vi "Topo & GridSpectr_DriftCorrection_v12.vi"(6 "Internal use":string, 7 "Grid param":T1 {"height (m)" format="%#_6p"; "width (m)" format="%#_6p"; "center Y (m)" format="%#_6p"; "center X (m)" format="%#_6p"}, 8 "Error in (no error)":errorcluster, 9 "Points Y/Index Y":i32, 10 "Points X/Index X":i32, 11 "Method":enum16{"init", "run", "end"}(ring)=enum."end") -> (0 "Error out":errorcluster)   [LabVIEW 2014]
doc: "Example of a measurement VI to be used in the \"Experiments on a Grid\" tool as external VI.\n\nThis example measure the topography and spectroscopy data. The spectroscopy measurements are taken on a subgrid. The data are saved to a sxm and a binary file.\n\n- Nanonis Programming Interface -"
uses:
  <userlib>/Nanonis Prog Interface V5/Scan/Grid/LinePatternGet.vi
  <userlib>/Nanonis Prog Interface V5/Scan/Grid/GridPatternGet.vi
  <userlib>/Nanonis Prog Interface V5/Scan/Grid/CloudPatternGet.vi
  <userlib>/Nanonis Prog Interface V5/Nanonis Prog Interface.lvlib
panel:
  in  "type":u16(ring)=1 items=["Line", "Grid", "Cloud"]
  in  "Lockin ON/OFF":bool
  in  "Correct Drift":bool=TRUE
  in  "Email when finished":string="cornelius.krull@monash.edu, dhaneesh.gopalakrishnan@monash.edu"
  in  "STS z offset":dbl format="%#_6p"
  out "ETA":timestamp=timestamp(3582621546.85837 s since 1904-01-01)
  out "remaining":dbl=19834.093046092985 format="%<%H:%M:%S>t"
  out "Progress":u8(slide)=5 scale=0.0..100.0 scale format="%#.1g"
  out "total Points":i32=576
  in  "preSTS delay [ms]":u32=3
  in  "STS Bias":dbl=-3.4 format="%#_6p"
  in  "Move Bias":dbl=-3.4 format="%#_6p"
  in  "Move Current":dbl=5e-11 format="%#_6p"
  in  "Imaging Bias":dbl=-3.4 format="%#_6p"
  in  "max applied Drift Correction":i32=20 min=1 max=100 step=1 format="%.0p"
  in  "Correlate":u16(ring) items=["first Frame", "successive Frames"]
  out "Topo Images taken":i32
  in  "Increment":i32=40
  in  "Threshold":i32=2 min=1 step=1
  in  "tip Speed (m/s)":sgl=1e-08 format="%.2p"
  out "X drift":i32
  out "Y drift":i32
  out "Last Drift detected":i32
  in  "MaxImagesBack":i32=2
  in  "Channel index (0-23)":u8(ring) items=["Current"=0, "Z (m)"=14]
  in  "File name":string="DCA_cluster_STS_Grid"
  in  "STS Current":dbl=5e-11 format="%#_6p"
  in  "Imaging Current":dbl=5e-11 format="%#_6p"
  in  "zdrift \nDuration (s)":dbl
  in  "Correct z drift":bool
  out "Status":string="finishing"
  in  "Drift correction Pixels":i32=256 caption="Topo Pixels"
  out "Y Offset":dbl format="%#_6p"
  out "X Offset":dbl format="%#_6p"
  out "Points taken":dbl=30.0
  in  "Drift Correction every":i32=40
  in  "Y subgrid spacing":u16=1
  in  "X subgrid spacing":u16=1
  # "GRID points"
  # "Increase this if no Drift was detected for \na certain number of images"
  # "%"
  # "time (HH:MM:SS)"
  # "images back"
  # "% of image size"
  # "RUN smart tilt before starting the GRID | Img Angle = 0"
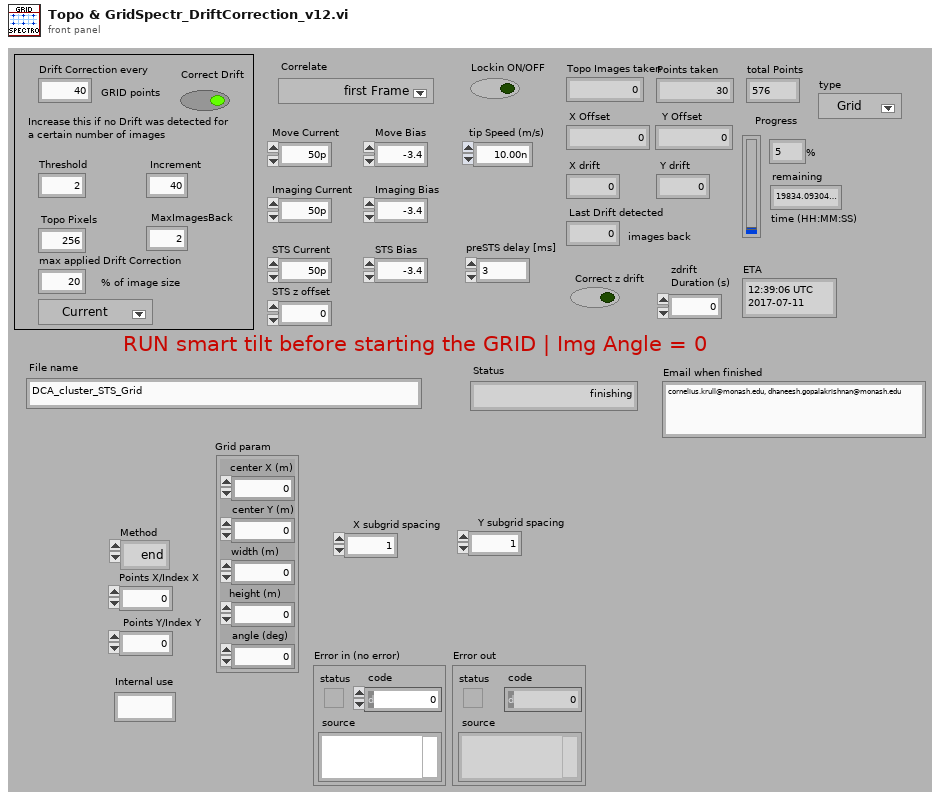
[diagram p1: front panel]
types:
  T1 = cluster{"center X (m)":sgl, "center Y (m)":sgl, "width (m)":sgl, "height (m)":sgl, "angle (deg)":sgl}
  T2 = cluster{"Drift correction Pixels":i32, "Imaging Current":dbl, "STS Current":dbl, "MaxImagesBack":i32, "tip Speed (m/s)":sgl, "Threshold":i32, "Increment":i32, "Correlate":u16, "max applied Drift Correction":i32, "Imaging Bias":dbl, "Move Current":dbl, "Move Bias":dbl, "STS Bias":dbl, "preSTS delay [ms]":u32, "STS z offset":dbl, "Correct Drift":bool, "Lockin ON/OFF":bool}
  T3 = cluster{"center X":sgl, "center Y":sgl, "angle":sgl, "width":sgl, "height":sgl, "# pixels":i32, "# lines":i32}
  T4 = cluster{"Name":string, "Calibration":sgl, "Offset":sgl, "Channel index":i32}[]
  T5 = cluster{"up/down":bool, "time/line":sgl, "start time":timestamp, "end time":timestamp}
  T6 = cluster{"Z averaging time (s)":sgl, "Z offset (m)":sgl, "Initial settling time (s)":sgl}
  T7 = cluster{"Max. slew rate (V/s)":sgl, "Settling time (s)":sgl, "Integration time (s)":sgl}
  T8 = cluster{"End settling time (s)":sgl, "Z control time (s)":sgl}
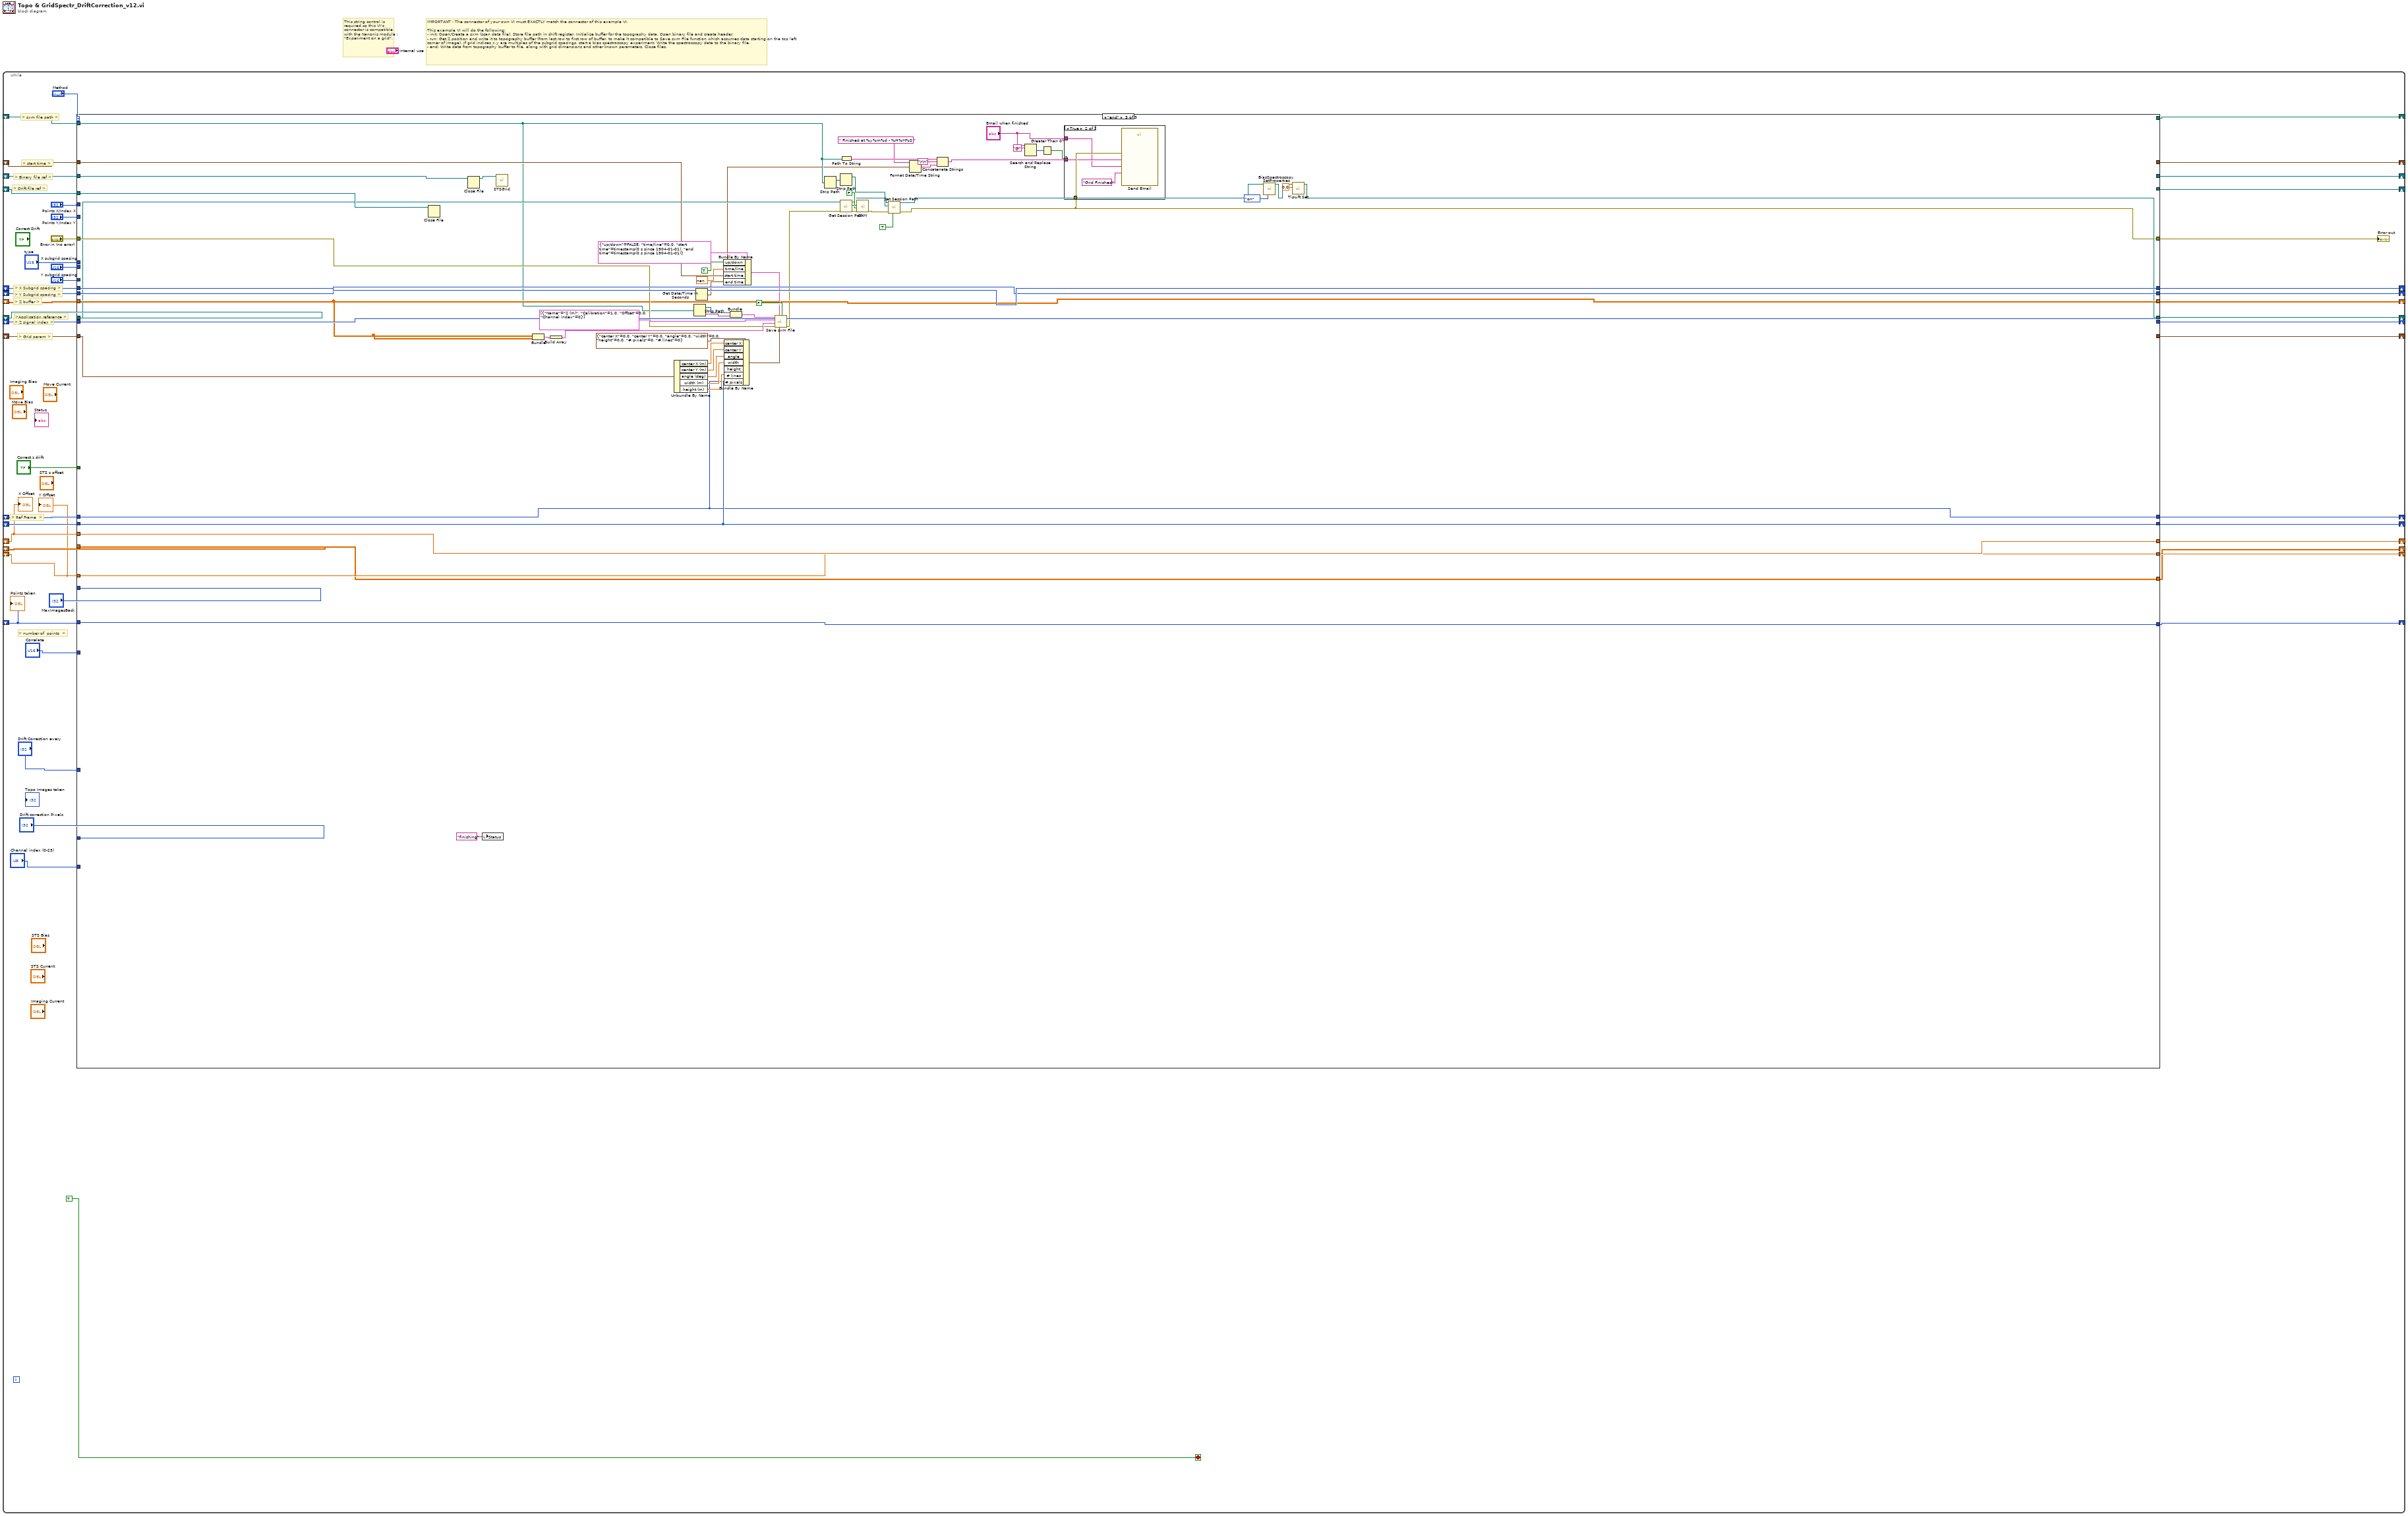
[diagram p0: block diagram]
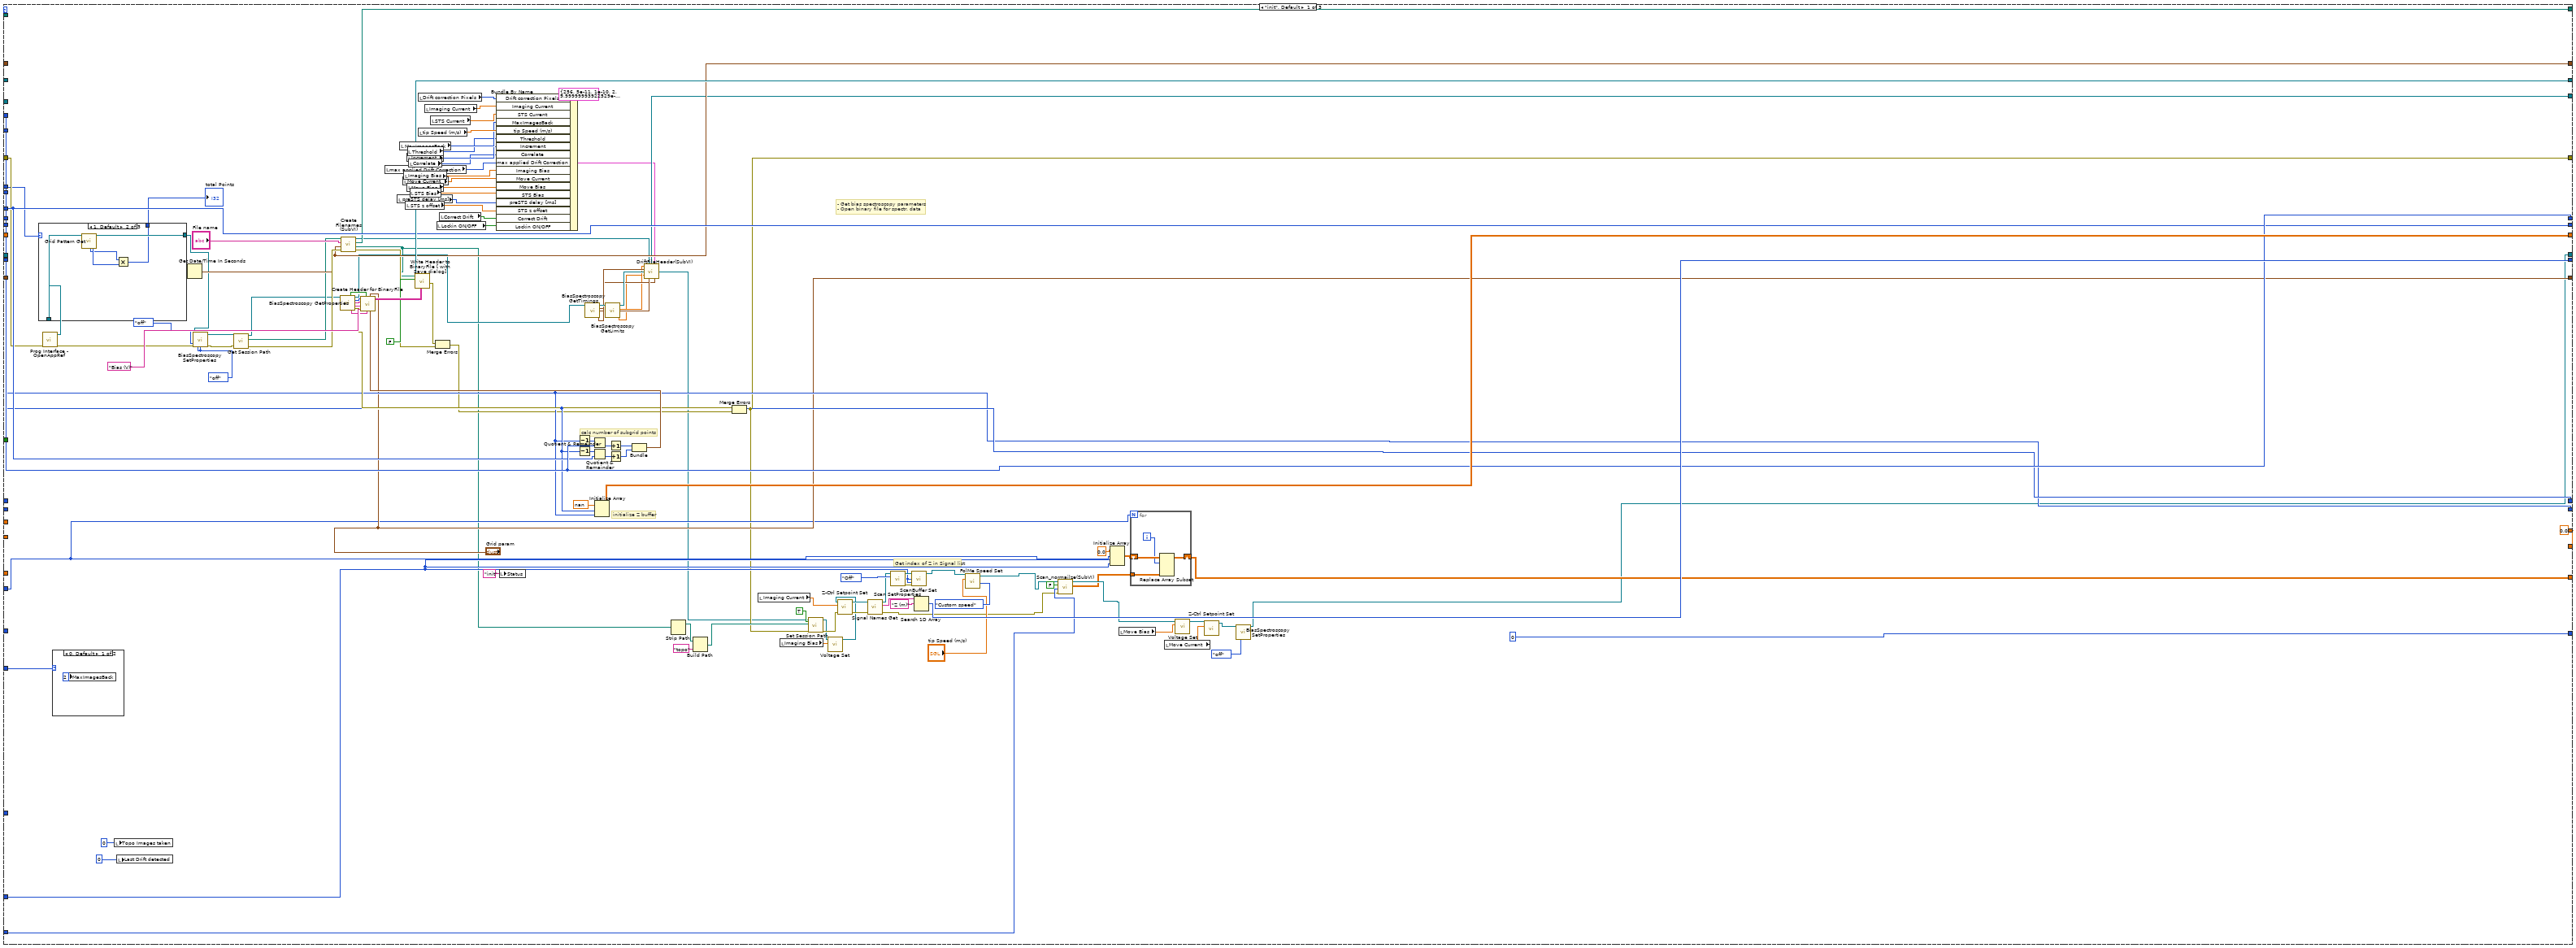
[diagram p2: hidden frame]
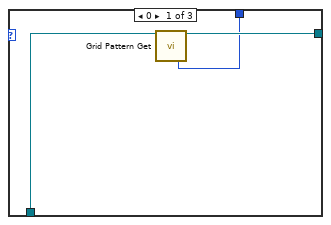
[diagram p3: hidden frame]
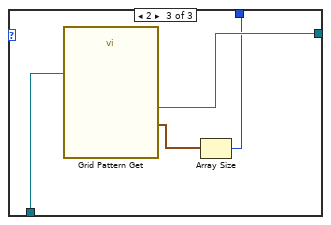
[diagram p4: hidden frame]
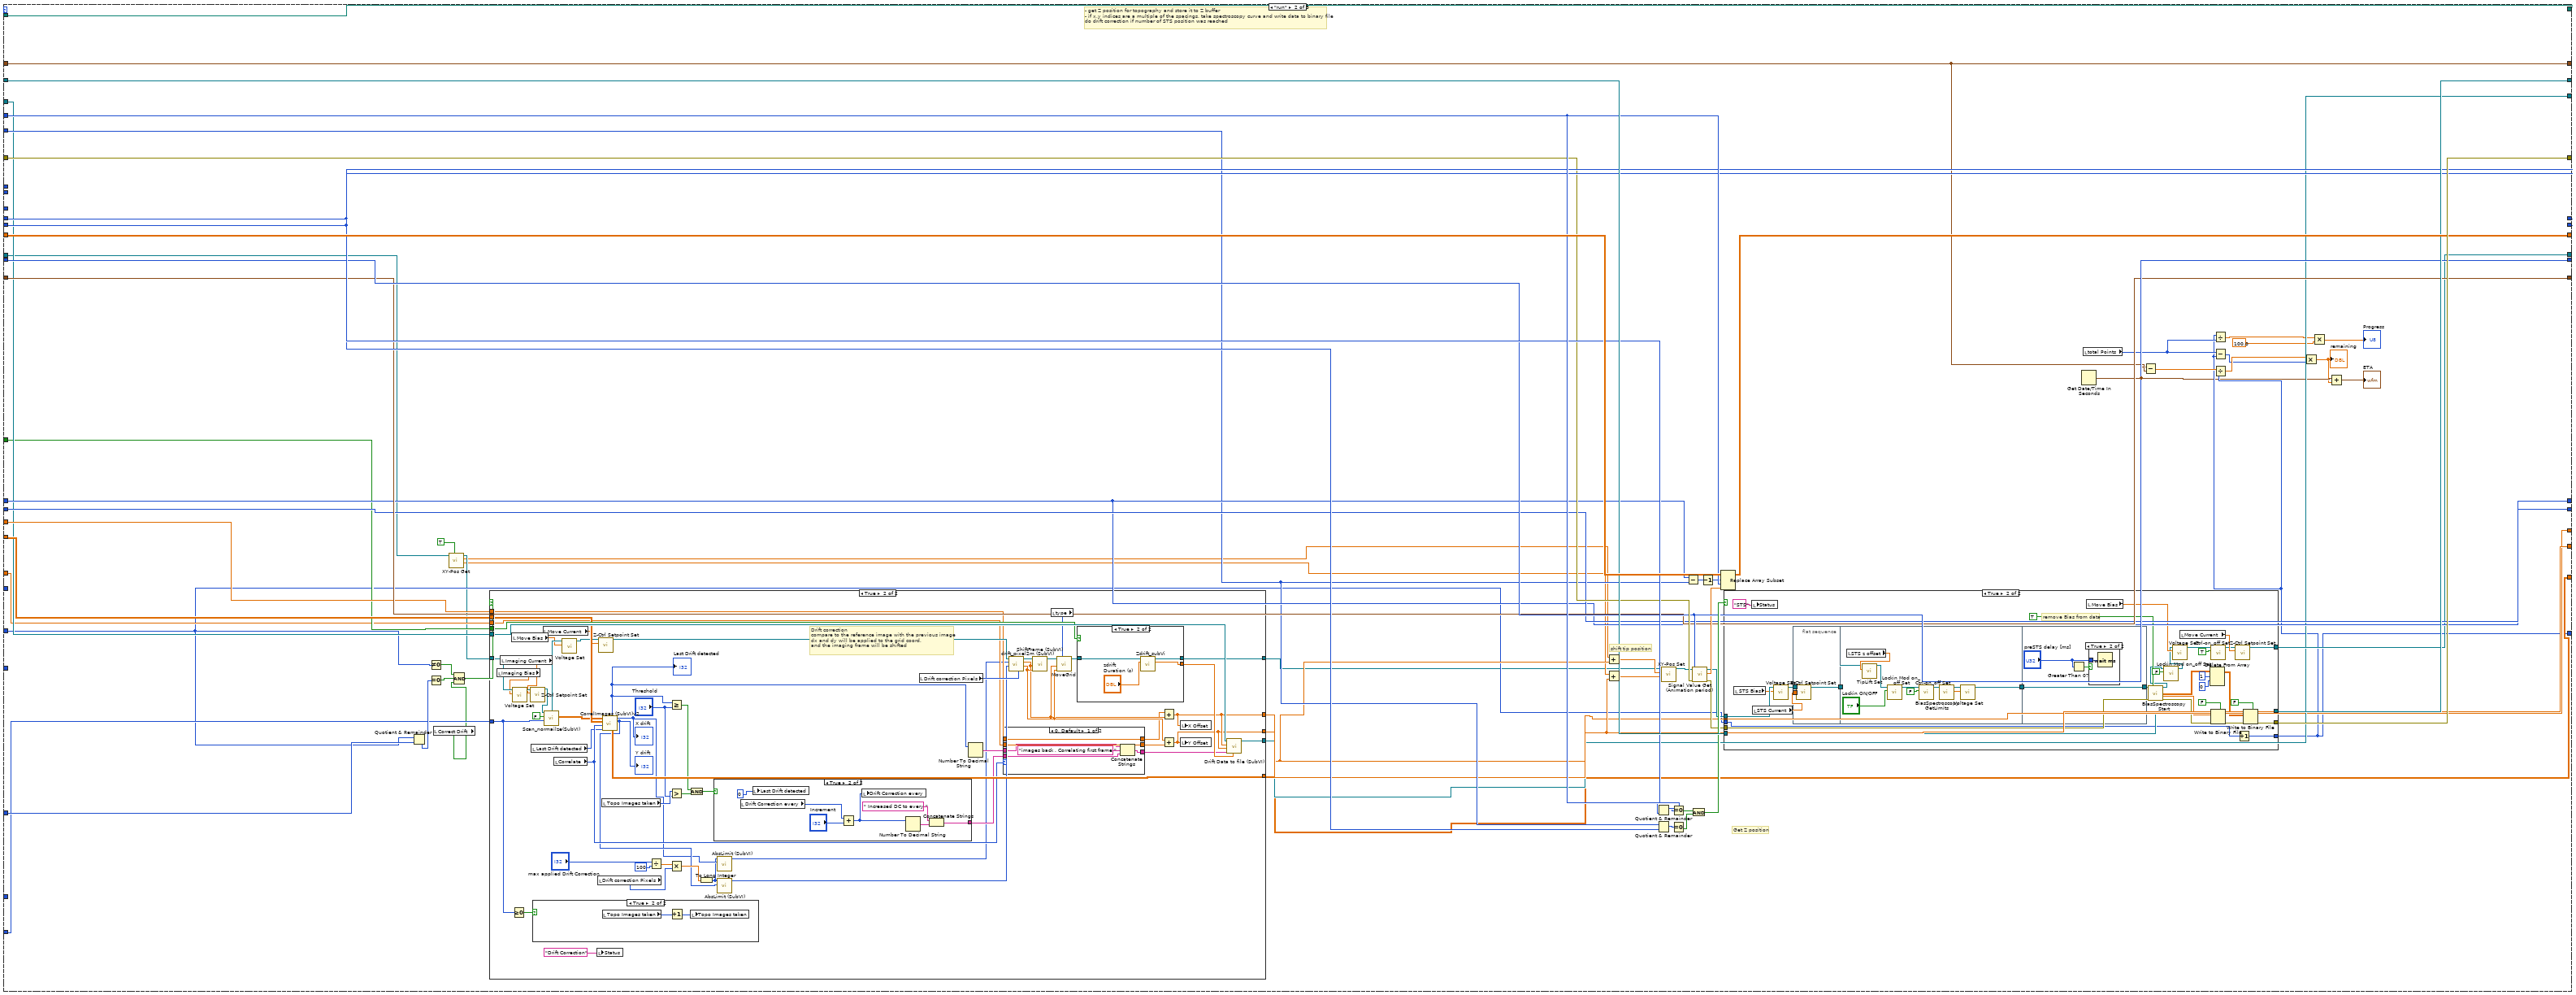
[diagram p6: hidden frame]
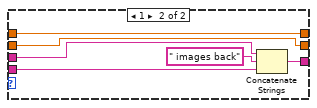
[diagram p8: hidden frame]
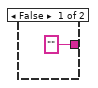
[diagram p10: hidden frame]
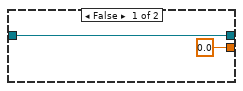
[diagram p11: hidden frame]
diagram:
  # "This string control is required so this VI's connector is compatible with the Nanonis module : \"Experiment on a grid\"."
  # "IMPORTANT : The connector of your own VI must EXACTLY match the connector of this example VI.\n\nThis example VI will do the following:\n- init: Open/Create a sxm (scan data file). Store file path in shift register. Initialize buffer for the topography data. Open binary file and create header.\n- run: Get Z position and write it to topography buffer (from last row to first row of buffer, to make it compatible to Save sxm File function which assumes data starting on the top left corner of image). If grid indices x,y are multiples of the subgrid spacings, start a bias spectroscopy experiment. Write the spectroscopy data to the binary file.\n- end: Write data from topography buffer to file, along with grid dimensions and other known parameters. Close files."
  n1 = while {
    shift-right: [w22] -> _
    shift-left: _ -> [w45]
    shift-right: [w40] -> _
    shift-left: _ -> [w39]
    shift-right: [w37] -> _
    shift-left: _ -> [w38]
    shift-right: [w36] -> _
    shift-left: _ -> [w35]
    shift-right: [w29] -> _
    shift-left: _ -> [w31]
    shift-right: [w30] -> _
    shift-left: _ -> [w32]
    shift-right: [w28] -> _
    shift-left: _ -> [w27]
    shift-right: [w26] -> _
    shift-left: _ -> [w25]
    shift-right: [w24] -> _
    shift-left: _ -> [w23]
    shift-right: [w21] -> _
    shift-left: _ -> [w20]
    shift-right: [w19] -> _
    shift-left: _ -> [w18]
    shift-right: [w17] -> _
    shift-left: _ -> [w10]
    shift-right: [w16] -> _
    shift-left: _ -> [w9]
    shift-right: [w15] -> _
    shift-left: _ -> [w12]
    shift-right: [w14] -> _
    shift-left: _ -> [w11]
    shift-right: [w7] -> _
    shift-left: _ -> [w6]
    stop <- TRUE stop-if-true
    # "> Drift file ref >"
    # "> number of  points  >"
    # "> Ref Frame  >"
    # "> Grid param >"
    # "> start time >"
    # ">Application reference >"
    # "> Y Subgrid spacing >"
    # "> X Subgrid spacing >"
    # "> Z signal index >"
    # "> Binary file ref >"
    # "> Z buffer >"
    # "> sxm file path >"
    n2 = case shown="\"end\"" "Method" {
      tunnel: [w128 w247 _] -> w22
      tunnel: w45 -> [_ w247 w412]
      tunnel: "Error in (no error)" -> [w130 w233 w439]
      tunnel: [w52 w246 w394] -> w43
      tunnel: "Points X/Index X" -> [w142 w241 _]
      tunnel: "Points Y/Index Y" -> [w143 w226 _]
      tunnel: [w166 w244 w428] -> w40
      tunnel: w39 -> [_ w245 w428]
      tunnel: w38 -> [_ w243 w421]
      tunnel: [w158 w242 _] -> w37
      tunnel: [w156 w231 w453] -> w36
      tunnel: w35 -> [_ w231 w453]
      tunnel: "X subgrid spacing" -> [w155 _ _]
      tunnel: "Y subgrid spacing" -> [w154 _ _]
      tunnel: w32 -> [_ w235 w452]
      tunnel: w31 -> [_ w234 w451]
      tunnel: [w155 w235 w452] -> w30
      tunnel: [w154 w234 w451] -> w29
      tunnel: [w92 w219 w399] -> w28
      tunnel: w27 -> [_ w202 w416]
      tunnel: ["Grid param" w229 _] -> w26
      tunnel: w25 -> [_ w229 w438]
      tunnel: [w127 w192 _] -> w24
      tunnel: w23 -> [_ w192 w446]
      tunnel: [w143 w227 w429] -> w21
      tunnel: w20 -> [_ w227 w429]
      tunnel: [w142 w228 w430] -> w19
      tunnel: w18 -> [_ w228 w430]
      tunnel: [w139 w209 w427] -> w17
      tunnel: [w139 w214 w425] -> w16
      tunnel: [w123 w208 w422] -> w15
      tunnel: [0 w190 w426] -> w14
      tunnel: w11 -> [_ w205 w426]
      tunnel: "Drift Correction every" -> [_ w222 _]
      tunnel: w12 -> [_ w213 w422]
      tunnel: w10 -> [_ w220 w427]
      tunnel: w9 -> [_ w206 w425]
      tunnel: "Drift correction Pixels" -> [w122 _ _]
      tunnel: [w87 w211 _] -> w7
      tunnel: w6 -> [_ w212 w423]
      tunnel: "Correct z drift" -> [_ w210 _]
      tunnel: "Channel index (0-23)" -> [w61 w207 _]
      tunnel: "MaxImagesBack" -> [w121 _ _]
      tunnel: "Correlate" -> [w103 _ _]
      tunnel: "type" -> [w55 _ _]
      frame "init", Default {
        w89 = enum16{"no change", "on", "off"}."off" ("Save dialog")
        w139 = 0.0
        # "- Get bias spectroscopy parameters\n- Open binary file for spectr. data"
        # "initialize Z buffer"
        # "calc number of subgrid points"
        # "Get index of Z in Signal list"
        n3 = call <userlib>:"Prog Interface - OpenAppRef.vi"("Error in (no error)"=w130) -> ("Error out"=w109:errorcluster, "Application reference"=w94:refnum<vi>)  [unwired: 5 in]
        n4 = case shown="1, Default" w55 {
          tunnel: w94 -> [w169 w174 w178]
          tunnel: [w168 w173 w177] -> w93
          tunnel: [w167 w170 w175] -> w54
          frame 0 {
            n5 = call-poly <userlib>:"Grid Pattern Get.vi"("Application ref in"=w169) -> ("Points"=w167:i32, "Application ref out"=w168:refnum<vi>)  [unwired: 12 in, 5 out]
          }
          frame 1, Default {
            n6 = call-poly <userlib>:"Grid Pattern Get.vi"("Application ref in"=w174) -> ("Points Y"=w171:i32, "Points X"=w172:i32, "Application ref out"=w173:refnum<vi>)  [unwired: 10 in, 6 out]
            n7 = Multiply(x=w171, y=w172) -> (x*y=w170:i32)
          }
          frame 2 {
            n8 = call-poly <userlib>:"Grid Pattern Get.vi"("Application ref in"=w178) -> ("Application ref out"=w177:refnum<vi>, "Cloud data"=w176:cluster{"X":sgl, "Y":sgl}[])  [unwired: 16 in, 1 out]
            n9 = Array Size(array=w176) -> (size(s)=w175:i32)
          }
        }
        "total Points" <- w54
        n10 = case shown="0, Default" w103 {
          frame 0, Default {
            n11 = local write "MaxImagesBack"(2 ("StepsBack")) -> ()
          }
          frame 1 {
          }
        }
        n12 = local write "Topo Images taken"(0 ("Images taken")) -> ()
        n13 = local write "Last Drift detected"(0 ("Last Drift detected")) -> ()
        n14 = Get Date/Time In Seconds() -> (seconds since 1Jan1904=w127:timestamp)
        n15 = call <userlib>:"BiasSpectroscopy SetProperties.vi"("Application ref in"=w93, "Autosave (no change)"=enum16{"no change", "on", "off"}."off", "Error in (no error)"=w109, "Z-Controller hold (no change)"=w89, "Save dialog"=w89) -> ("Application ref out"=w106:refnum<vi>, "Error out"=w105:errorcluster)  [unwired: 9 in]
        n16 = call <userlib>:"Get Session Path.vi"("error in (no error)"=w105, "Application ref in"=w106) -> ("error out"=w129:errorcluster, "Session path"=w113:path, "Application ref out"=w107:refnum<vi>)  [unwired: 7 in]
        n17 = call <userlib>:"BiasSpectroscopy GetProperties.vi"("Application ref in"=w107) -> ("Backward sweep"=w162:bool, "Application ref out"=w116:refnum<vi>, "Number of points"=w145:i32, "Channels"=w144:string[], "Parameters"=w160:string[], "Fixed parameters"=w147:string[], "Error out"=w159:errorcluster)  [unwired: 6 in, 2 out]
        n18 = call "Create Filenames (SubVI).vi"("error in (no error)"=w129, "seconds since 1Jan1904"=w127, "File name"="File name", "Session path"=w113) -> ("error out"=w117:errorcluster, "binFilePath"=w110:path, "topoFilePath"=w128:path, "Drift File out"=w88:refnum<file>)  [unwired: 4 in]
        n19 = local read "max applied Drift Correction"() -> (w69:i32)
        n20 = local read "preSTS delay [ms]"() -> (w64:u32)
        n21 = local read "MaxImagesBack"() -> (w73:i32)
        n22 = local read "Move Current"() -> (w67:dbl)
        n23 = local read "Imaging Bias"() -> (w68:dbl)
        n24 = local read "STS z offset"() -> (w63:dbl)
        n25 = local read "Increment"() -> (w71:i32)
        n26 = local read "Move Bias"() -> (w66:dbl)
        n27 = local read "Threshold"() -> (w72:i32)
        n28 = local read "Correlate"() -> (w70:u16)
        n29 = local read "STS Bias"() -> (w65:dbl)
        n30 = local read "Drift correction Pixels"() -> (w78:i32)
        n31 = local read "tip Speed (m/s)"() -> (w75:sgl)
        n32 = local read "Imaging Current"() -> (w77:dbl)
        n33 = local read "STS Current"() -> (w76:dbl)
        n34 = local read "Lockin ON/OFF"() -> (w74:bool)
        n35 = local read "Correct Drift"() -> (w62:bool)
        n36 = Bundle By Name(cluster=T2 {"Drift correction Pixels"=256, "Imaging Current"=5e-11, "STS Current"=1e-10, "MaxImagesBack"=2, "tip Speed (m/s)"=1e-08, "Threshold"=2, "Increment"=64, "Correlate"=0, "max applied Drift Correction"=20, "Imaging Bias"=-0.02, "Move Current"=1.5e-11, "Move Bias"=-0.02, "STS Bias"=0.1, "preSTS delay [ms]"=1000, "STS z offset"=-1.7e-10, "Correct Drift"=TRUE, "Lockin ON/OFF"=TRUE} ("Drift Correction"), "Drift correction Pixels"=w78, "Imaging Current"=w77, "STS Current"=w76, "MaxImagesBack"=w73, "tip Speed (m/s)"=w75, "Threshold"=w72, "Increment"=w71, "Correlate"=w70, "max applied Drift Correction"=w69, "Imaging Bias"=w68, "Move Current"=w67, "Move Bias"=w66, "STS Bias"=w65, "preSTS delay [ms]"=w64, "STS z offset"=w63, "Correct Drift"=w62, "Lockin ON/OFF"=w74) -> (w80:T2)
        n37 = local write "Status"("init" ("Status")) -> ()
        n38 = Decrement(x=w142) -> (x-1=w153:i32)
        n39 = Decrement(x=w143) -> (x-1=w152:i32)
        n40 = call <userlib>:"BiasSpectroscopy GetTimings.vi"("Application ref in"=w116) -> ("Application ref out"=w120:refnum<vi>, "Initialization"=w83:T6, "Sweep Timing"=w84:T7, "End of Sweep"=w85:T8)  [unwired: 10 in, 1 out]
        n41 = Quotient & Remainder(x=w153, y=w155) -> (floor(x/y)=w151:i32)  [unwired: 1 out]
        n42 = Quotient & Remainder(x=w152, y=w154) -> (floor(x/y)=w150:i32)  [unwired: 1 out]
        n43 = Initialize Array(sgl nan ("element"), w143, w142) -> (w166:sgl[][])
        n44 = call <userlib>:"BiasSpectroscopy GetLimits.vi"("Application ref in"=w120) -> ("End value (V)"=w81:sgl, "Start value (V)"=w82:sgl, "Application ref out"=w86:refnum<vi>)  [unwired: 5 in, 1 out]
        n45 = Increment(x=w151) -> (x+1=w149:i32)
        n46 = Increment(x=w150) -> (x+1=w148:i32)
        n47 = Bundle(w149, w148) -> (w161:cluster{i32, i32})  [unwired: 1 in]
        n48 = call <userlib>:"Create Header for BinaryFile.vi"("Grid points"=w161, "Grid param"="Grid param", "Fixed parameters"=w147, "Backward sweep"=w162, "Sweep signal"="Bias (V)" ("Sweep Signal"), "Parameters"=w160, "Channels"=w144, "Points per sweep"=w145) -> ("Header (fixed attributes)"=w164:string[][])  [unwired: 3 in]
        n49 = call <userlib>:"Write Header to BinaryFile [ with Save dialog].vi"("Fixed Attributes"=w164, "Show Dialog? (T)"=FALSE, "Filename"=w110) -> ("Error out"=w118:errorcluster, "File ref"=w158:refnum<file>)  [unwired: 5 in, 2 out]
        n50 = Merge Errors(w118, w117) -> (w119:errorcluster)
        n51 = call "DriftFileHeader(SubVI).vi"("Start value (V)"=w82, "Byte Stream File in"=w88, "Drift Correction"=w80, "End of Sweep"=w85, "Application ref in"=w86, "End value (V)"=w81, "Sweep Timing"=w84, "Initialization"=w83) -> ("Byte Stream File out"=w87:refnum<file>, "Application ref out"=w49:refnum<vi>)  [unwired: 6 in]
        n52 = Strip Path(path=w110) -> (stripped path=w112:path)  [unwired: 1 out]
        n53 = Build Path(base path=w112, name or relative path="topo") -> (appended path=w53:path)
        n54 = Merge Errors(w159, w119) -> (w52:errorcluster)
        n55 = local read "Imaging Current"() -> (w95:dbl)
        n56 = local read "Imaging Bias"() -> (w96:dbl)
        n57 = call <userlib>:"Set Session Path.vi"("Save settings to previous? (False)"=TRUE, "error in (no error)"=w52, "Session Folder"=w53, "Application ref in"=w49) -> ("error out"=w51:errorcluster, "Application ref out"=w48:refnum<vi>)  [unwired: 6 in]
        n58 = call <userlib>:"Voltage Set.vi"("Bias (V)"=w96, "Application ref in"=w48) -> ("Application ref out"=w99:refnum<vi>)  [unwired: 8 in, 1 out]
        n59 = call <userlib>:"Z-Ctrl Setpoint Set.vi"("error in (no error)"=w51, "Z Controller setpoint"=w95, "Application ref in"=w99) -> ("error out"=w131:errorcluster, "Application ref out"=w132:refnum<vi>)  [unwired: 7 in]
        n60 = call <userlib>:"Signal Names Get.vi"("error in (no error)"=w131, "Application ref in"=w132) -> ("error out"=w58:errorcluster, "Signals Names"=w146:string[], "Application ref out"=w135:refnum<vi>)  [unwired: 5 in]
        n61 = call <userlib>:"Scan SetProperties.vi"("Application ref in"=w135, "Continuous scan"=enum16{"No change", "On", "Off"}."Off") -> ("Application ref out"=w137:refnum<vi>, "Error out"=w136:errorcluster)  [unwired: 12 in]
        n62 = call <userlib>:"ScanBuffer Set.vi"("Application ref in"=w137, "Pixels"=w122, "Lines"=w122, "error in (no error)"=w136) -> ("Application ref out"=w101:refnum<vi>)  [unwired: 10 in, 1 out]
        n63 = Search 1D Array(1D array=w146, element="Z (m)") -> (index of element=w156:i32)  [unwired: 1 in]
        n64 = call <userlib>:"FolMe Speed Set.vi"("Speed Setting (Custom)"=enum32{"Scan speed", "Custom speed"}."Custom speed", "Speed (m/s)"="tip Speed (m/s)", "Application ref in"=w101) -> ("Application ref out"=w60:refnum<vi>)  [unwired: 5 in, 1 out]
        n65 = call "Scan_normailze(SubVI).vi"("error in (no error)"=w58, "Channel index (0-23)"=w61, "Normalization"=FALSE ("Boolean"), "Application in"=w60) -> ("Array"=w57:dbl[][], "Application out"=w59:refnum<vi>)  [unwired: 5 in, 1 out]
        n66 = Initialize Array(0.0 ("element"), w121, w122, w122) -> (w124:dbl[][][])
        n67 = local read "Move Bias"() -> (w98:dbl)
        n68 = for {
          N: w121 -> [_]
          tunnel: w57 -> [w182]
          shift-right: [w181] -> w123
          shift-left: w124 -> [w183]
          i -> [w180]
          n69 = Replace Array Subset(array=w183, new element=w182, index (dim 0)=w180) -> (w181:dbl[][][])  [unwired: 2 in]
        }
        n70 = local read "Move Current"() -> (w97:dbl)
        n71 = call <userlib>:"Voltage Set.vi"("Bias (V)"=w98, "Application ref in"=w59) -> ("Application ref out"=w100:refnum<vi>)  [unwired: 8 in, 1 out]
        n72 = call <userlib>:"Z-Ctrl Setpoint Set.vi"("Z Controller setpoint"=w97, "Application ref in"=w100) -> ("Application ref out"=w91:refnum<vi>)  [unwired: 8 in, 1 out]
        n73 = call <userlib>:"BiasSpectroscopy SetProperties.vi"("Application ref in"=w91, "Z-Controller hold (no change)"=enum16{"no change", "on", "off"}."off") -> ("Application ref out"=w92:refnum<vi>)  [unwired: 12 in, 1 out]
      }
      frame "run" {
        # "shift tip position"
        # "Get Z position"
        # "- get Z position for topography and store it to Z buffer\n- if x,y indices are a multiple of the spacings, take spectroscopy curve and write data to binary file\ndo drift correction if number of STS position was reached"
        n74 = Quotient & Remainder(x=w205, y=w222) -> (x-y*floor(x/y)=w223:i32)  [unwired: 1 out]
        n75 = Not Equal To 0?(x=w205) -> (x != 0?=w203:bool)
        n76 = Equal To 0?(x=w223) -> (x = 0?=w221:bool)
        n77 = local read "Correct Drift"() -> (w184:bool)
        n78 = call <userlib>:"XY-Pos Get.vi"("Wait for newest data (F=False)"=TRUE, "Application ref in"=w202) -> ("Y (m)"=w198:sgl, "X (m)"=w199:sgl, "Application ref out"=w201:refnum<vi>)  [unwired: 5 in, 1 out]
        n79 = Compound Arithmetic op=AND(w203, w221, w184) -> (w204:bool)
        n80 = case shown="True" w204 {
          tunnel: w201 -> [w252 w262]
          tunnel: [w252 w304] -> w197
          tunnel: w213 -> [w249 w299]
          tunnel: [w251 w302] -> w209
          tunnel: [w250 w301] -> w214
          tunnel: w220 -> [w251 w278]
          tunnel: w206 -> [w250 w276]
          tunnel: [w249 w295] -> w208
          tunnel: w212 -> [w248 w307]
          tunnel: [w248 w306] -> w211
          tunnel: w210 -> [_ w303]
          tunnel: w207 -> [_ w282]
          frame False {
          }
          frame True {
            # "Drift correction \ncompare to the reference image with the previous image \ndx and dy will be applied to the grid coord, \nand the imaging frame will be shifted"
            n81 = local read "Imaging Bias"() -> (w260:dbl)
            n82 = local read "Imaging Current"() -> (w259:dbl)
            n83 = local read "Move Bias"() -> (w256:dbl)
            n84 = Greater Or Equal To 0?(x=w282) -> (x >= 0?=w281:bool)
            n85 = call <userlib>:"Voltage Set.vi"("Bias (V)"=w260, "Application ref in"=w262) -> ("Application ref out"=w261:refnum<vi>)  [unwired: 8 in, 1 out]
            n86 = call <userlib>:"Z-Ctrl Setpoint Set.vi"("Z Controller setpoint"=w259, "Application ref in"=w261) -> ("Application ref out"=w300:refnum<vi>)  [unwired: 8 in, 1 out]
            n87 = local read "Last Drift detected"() -> (w273:i32)
            n88 = case shown="True" w281 {
              frame False {
              }
              frame True {
                n89 = local read "Topo Images taken"() -> (w322:i32)
                n90 = Increment(x=w322) -> (x+1=w321:i32)
                n91 = local write "Topo Images taken"(w321) -> ()
              }
            }
            n92 = local read "Move Current"() -> (w255:dbl)
            n93 = call "Scan_normailze(SubVI).vi"("Channel index (0-23)"=w282, "Normalization"=FALSE ("Boolean"), "Application in"=w300) -> ("Array"=w296:dbl[][], "Application out"=w257:refnum<vi>)  [unwired: 6 in, 1 out]
            n94 = local read "Correlate"() -> (w279:u16)
            n95 = call <userlib>:"Voltage Set.vi"("Bias (V)"=w256, "Application ref in"=w257) -> ("Application ref out"=w258:refnum<vi>)  [unwired: 8 in, 1 out]
            n96 = local write "Status"("Drift Correction" ("Status")) -> ()
            n97 = local read "Drift correction Pixels"() -> (w270:i32)
            n98 = call <userlib>:"Z-Ctrl Setpoint Set.vi"("Z Controller setpoint"=w255, "Application ref in"=w258) -> ("Application ref out"=w291:refnum<vi>)  [unwired: 8 in, 1 out]
            n99 = local read "Topo Images taken"() -> (w284:i32)
            n100 = call "CorrelImages (SubVI)v2.vi"("last drift detected"=w273, "Correlate"=w279, "Ref Array"=w299, "New Image"=w296) -> ("Y drift"=w267:i32, "X drift"=w264:i32, "Ref Array out"=w295:dbl[][][], "Queue Steps"=w280:i32)  [unwired: 4 in]
            "X drift" <- w264
            "Y drift" <- w267
            "Last Drift detected" <- w280
            n101 = Divide(x="max applied Drift Correction", y=100) -> (x/y=w269:dbl)
            n102 = Greater Or Equal?(x=w280, y="Threshold") -> (x >= y?=w286:bool)
            n103 = Greater?(x=w284, y="Threshold") -> (0:w283:bool)
            n104 = Multiply(x=w269, y=w270) -> (x*y=w271:dbl)
            n105 = And(x=w286, y=w283) -> (x .and. y?=w285:bool)
            n106 = To Long Integer(number=w271) -> (32bit integer=w263:i32)
            n107 = case shown="True" w285 {
              tunnel: ["" w326] -> w287
              frame False {
              }
              frame True {
                n108 = local read "Drift Correction every"() -> (w325:i32)
                n109 = local write "Last Drift detected"(0 ("Last Drift detected")) -> ()
                n110 = Add(x=w325, y="Increment") -> (x+y=w329:i32)
                n111 = local write "Drift Correction every"(w329) -> ()
                n112 = Number To Decimal String(number=w329) -> (decimal integer string=w328:string)  [unwired: 1 in]
                n113 = Concatenate Strings(" Increased DC to every " ("string"), w328) -> (w326:string)
              }
            }
            n114 = call "AbsLimit (SubVI).vi"("in"=w264, "Abslimt"=w263) -> ("Numeric out"=w266:i32)  [unwired: 9 in]
            n115 = call "AbsLimit (SubVI).vi"("in"=w267, "Abslimt"=w263) -> ("Numeric out"=w265:i32)  [unwired: 9 in]
            n116 = local read "Drift correction Pixels"() -> (w292:i32)
            n117 = Number To Decimal String(number=w280) -> (decimal integer string=w298:string)  [unwired: 1 in]
            n118 = case shown="0, Default" w279 {
              tunnel: w298 -> [w309 w320]
              tunnel: [w314 w319] -> w297
              tunnel: w287 -> [w312 w317]
              tunnel: w278 -> [w310 w316]
              tunnel: [w310 w316] -> w277
              tunnel: w276 -> [w311 w315]
              tunnel: [w311 w315] -> w275
              frame 0, Default {
                n119 = Concatenate Strings(w309, "images back , Correlating first frame " ("string"), w312) -> (w314:string)
              }
              frame 1 {
                n120 = Concatenate Strings(w320, " images back" ("string"), w317) -> (w319:string)
              }
            }
            n121 = call "drift_pixel2m (SubVI).vi"("Application in"=w291, "X drift"=w266, "Y drift"=w265, "Drift correction Pixels"=w292) -> ("Application out"=w290:refnum<vi>, "x drift"=w288:sgl, "y drift"=w289:sgl)  [unwired: 2 in, 1 out]
            n122 = call "ShiftFrame (SubVI).vi"("Y shift"=w289, "X shift"=w288, "Application in"=w290) -> ("Application out"=w294:refnum<vi>)  [unwired: 8 in]
            n123 = local read "type"() -> (w253:u16)
            n124 = call "MoveGrid.vi"("type"=w253, "y"=w289, "x"=w288, "Application ref in"=w294) -> ("Application ref out"=w293:refnum<vi>)  [unwired: 6 in, 1 out]
            n125 = case shown="True" w303 {
              tunnel: [0.0 ("z drift") w336] -> w305
              tunnel: w293 -> [w331 w335]
              tunnel: [w331 w334] -> w304
              frame False {
              }
              frame True {
                n126 = call "Zdrift_subVi.vi"("Duration"="zdrift \nDuration (s)", "Application in"=w335) -> ("z drift"=w336:dbl, "Application out"=w334:refnum<vi>)  [unwired: 7 in, 1 out]
              }
            }
            n127 = Add(x=w277, y=w288) -> (x+y=w302:dbl)
            n128 = Add(x=w289, y=w275) -> (x+y=w301:dbl)
            n129 = local write "X Offset"(w302) -> ()
            n130 = local write "Y Offset"(w301) -> ()
            n131 = call "Drift Data to file (SubVI).vi"("z drift"=w305, "Comment"=w297, "y Drift"=w301, "X drift"=w302, "Byte Stream File in"=w307) -> ("Byte Stream File out"=w306:refnum<file>)  [unwired: 6 in]
          }
        }
        n132 = Add(x=w199, y=w209) -> (x+y=w216:dbl)
        n133 = Add(x=w198, y=w214) -> (x+y=w215:dbl)
        n134 = Quotient & Remainder(x=w241, y=w235) -> (x-y*floor(x/y)=w240:i32)  [unwired: 1 out]
        n135 = Quotient & Remainder(x=w226, y=w234) -> (x-y*floor(x/y)=w239:i32)  [unwired: 1 out]
        n136 = call <userlib>:"XY-Pos Set.vi"("Y (m)"=w215, "X (m)"=w216, "Application ref in"=w197) -> ("Application ref out"=w217:refnum<vi>)  [unwired: 5 in, 1 out]
        n137 = Equal To 0?(x=w240) -> (x = 0?=w238:bool)
        n138 = Equal To 0?(x=w239) -> (x = 0?=w237:bool)
        n139 = Subtract(x=w227, y=w226) -> (x-y=w225:i32)
        n140 = And(x=w238, y=w237) -> (x .and. y?=w236:bool)
        n141 = call <userlib>:"Signal Value Get (Animation period).vi"("error in (no error)"=w233, "Signal index (0-47)"=w231, "Application ref in"=w217) -> ("error out"=w232:errorcluster, "Signal value"=w230:sgl, "Application ref out"=w218:refnum<vi>)  [unwired: 5 in]
        n142 = Decrement(x=w225) -> (x-1=w224:i32)
        n143 = Replace Array Subset(array=w245, new element=w230, index (row)=w224, index (col)=w241) -> (w244:sgl[][])
        n144 = case shown="True" w236 {
          tunnel: [w339 w360] -> w246
          tunnel: w243 -> [w340 w374]
          tunnel: [w340 w372] -> w242
          tunnel: w232 -> [w339 w371]
          tunnel: w218 -> [w338 w356]
          tunnel: [w338 w351] -> w219
          tunnel: [w337 w358] -> w190
          tunnel: w205 -> [w337 w359]
          frame False {
            # "Point indices aren't multiple of subgrid spacing\n=> no spectroscopy at this point"
          }
          frame True {
            # "remove Bias from data"
            n145 = local read "STS Bias"() -> (w353:dbl)
            n146 = local write "Status"("STS" ("Status")) -> ()
            n147 = local read "STS Current"() -> (w352:dbl)
            n148 = call <userlib>:"Voltage Set.vi"("Bias (V)"=w353, "Application ref in"=w356) -> ("Application ref out"=w355:refnum<vi>)  [unwired: 8 in, 1 out]
            n149 = flat-sequence {
              tunnel: w355 -> [w377]
              tunnel: w352 -> [w375]
              tunnel: [w376] -> w348
              tunnel: w348 -> [w380]
              tunnel: [w378] -> w347
              tunnel: [w390] -> w354
              tunnel: w347 -> [w390]
              frame #0 {
                n150 = call <userlib>:"Z-Ctrl Setpoint Set.vi"("Z Controller setpoint"=w375, "Application ref in"=w377) -> ("Application ref out"=w376:refnum<vi>)  [unwired: 8 in, 1 out]
              }
              frame #1 {
                n151 = local read "STS z offset"() -> (w383:dbl)
                n152 = call <userlib>:"TipLift Set.vi"("TipLift (m)"=w383, "Application ref in"=w380) -> ("Application ref out"=w379:refnum<vi>)  [unwired: 8 in, 1 out]
                n153 = call <userlib>:"Lockin Mod on_off Set.vi"("Lockin ON/OFF"="Lockin ON/OFF", "Application ref in"=w379) -> ("Application ref out"=w382:refnum<vi>)  [unwired: 8 in, 1 out]
                n154 = call <userlib>:"Ctrl-on_off Set.vi"("Z Controller ON/OFF"=FALSE, "Application ref in"=w382) -> ("Application ref out"=w385:refnum<vi>)  [unwired: 8 in, 1 out]
                n155 = call <userlib>:"BiasSpectroscopy GetLimits.vi"("Application ref in"=w385) -> ("Start value (V)"=w384:sgl, "Application ref out"=w386:refnum<vi>)  [unwired: 5 in, 2 out]
                n156 = call <userlib>:"Voltage Set.vi"("Bias (V)"=w384, "Application ref in"=w386) -> ("Application ref out"=w378:refnum<vi>)  [unwired: 8 in, 1 out]
              }
              frame #2 {
                n157 = Greater Than 0?(x="preSTS delay [ms]") -> (x > 0?=w388:bool)
                n158 = case shown="True" w388 {
                  tunnel: "preSTS delay [ms]" -> [_ w391]
                  frame False {
                  }
                  frame True {
                    n159 = Wait (ms)(milliseconds to wait=w391) -> ()  [unwired: 1 out]
                  }
                }
              }
            }
            n160 = local read "Move Bias"() -> (w350:dbl)
            n161 = call <userlib>:"BiasSpectroscopy Start.vi"("Application ref in"=w354, "Get data (F)"=TRUE ("Get Data (F)"), "Error in (no error)"=w371) -> ("Application ref out"=w343:refnum<vi>, "Data"=w370:sgl[][], "Parameters"=w369:sgl[], "Error out"=w362:errorcluster)  [unwired: 8 in, 1 out]
            n162 = call <userlib>:"Lockin Mod on_off Set.vi"("Lockin ON/OFF"=FALSE, "Application ref in"=w343) -> ("Application ref out"=w342:refnum<vi>)  [unwired: 8 in, 1 out]
            n163 = call <userlib>:"Voltage Set.vi"("Bias (V)"=w350, "Application ref in"=w342) -> ("Application ref out"=w345:refnum<vi>)  [unwired: 8 in, 1 out]
            n164 = local read "Move Current"() -> (w349:dbl)
            n165 = Delete From Array(array=w370, length=1, index (row)=0 ("index")) -> (array with subset deleted=w368:sgl[][])  [unwired: 1 in, 1 out]
            n166 = call <userlib>:"Ctrl-on_off Set.vi"("Z Controller ON/OFF"=TRUE, "Application ref in"=w345) -> ("Application ref out"=w344:refnum<vi>)  [unwired: 8 in, 1 out]
            n167 = Write to Binary File(file (use dialog)=w374, data=w369, error in=w362, 5:FALSE ("prepend array or string size? (T)")) -> (refnum out=w373:refnum<file>, error out=w361:errorcluster)  [unwired: 2 in, 1 out]
            n168 = call <userlib>:"Z-Ctrl Setpoint Set.vi"("Z Controller setpoint"=w349, "Application ref in"=w344) -> ("Application ref out"=w351:refnum<vi>)  [unwired: 8 in, 1 out]
            n169 = Increment(x=w359) -> (x+1=w358:i32)
            n170 = Write to Binary File(file (use dialog)=w373, data=w368, error in=w361, 5:FALSE ("prepend array or string size? (T)")) -> (refnum out=w372:refnum<file>, error out=w360:errorcluster)  [unwired: 2 in, 1 out]
          }
        }
        n171 = Get Date/Time In Seconds() -> (seconds since 1Jan1904=w187:timestamp)
        n172 = local read "total Points"() -> (w193:i32)
        n173 = Subtract(x=w187, y=w192) -> (x-y=w191:dbl)
        n174 = Divide(x=w190, y=w193) -> (x/y=w196:dbl)
        n175 = Subtract(x=w193, y=w190) -> (x-y=w188:i32)
        n176 = Divide(x=w191, y=w190) -> (x/y=w189:dbl)
        n177 = Multiply(x=w189, y=w188) -> (x*y=w186:dbl)
        "remaining" <- w186
        n178 = Multiply(x=w196, y=100.0) -> (x*y=→"Progress":dbl)
        n179 = Add(x=w187, y=w186) -> (x+y=→"ETA":timestamp)
      }
      frame "end" {
        n180 = Close File(refnum=w423) -> ()  [unwired: 1 in, 2 out]
        n181 = Close File(refnum=w421) -> (path=w420:path)  [unwired: 1 in, 1 out]
        n182 = local write "Status"("finishing" ("Status")) -> ()
        n183 = call "STSGrid.vi"("Binary Spectroscopy File"=w420) -> ()  [unwired: 11 in]
        n184 = Bundle(w428, w428) -> (w450:cluster{sgl[][], sgl[][]})  [unwired: 1 in]
        n185 = Build Array(w450) -> (w449:cluster{sgl[][], sgl[][]}[])
        n186 = Unbundle By Name(w438) -> ("center X (m)"=w436:sgl, "center Y (m)"=w435:sgl, "angle (deg)"=w434:sgl, "width (m)"=w433:sgl, "height (m)"=w432:sgl)
        n187 = Strip Path(path=w412) -> (stripped path=w442:path, name=w441:string)
        n188 = Get Date/Time In Seconds() -> (seconds since 1Jan1904=w408:timestamp)
        n189 = Bundle By Name(cluster=T5 {"up/down"=FALSE, "time/line"=0.0, "start time"=timestamp(0 s since 1904-01-01), "end time"=timestamp(0 s since 1904-01-01)} ("Scan param"), "up/down"=TRUE, "time/line"=sgl nan ("input 7"), "start time"=w446, "end time"=w408) -> (w445:T5)
        n190 = Bundle By Name(cluster=T3 {"center X"=0.0, "center Y"=0.0, "angle"=0.0, "width"=0.0, "height"=0.0, "# pixels"=0, "# lines"=0} ("Scanfield"), "center X"=w436, "center Y"=w435, "angle"=w434, "width"=w433, "height"=w432, "# lines"=w429, "# pixels"=w430) -> (w431:T3)
        n191 = Bundle("stripped path"=w442, "name"=w441) -> (w440:cluster{"stripped path":path, "name":string})  [unwired: 1 in]
        n192 = call <userlib>:"Save sxm File.vi"("Auto file naming? (T)"=FALSE, "Scanfield"=w431, "Scan param"=w445, "error in (no error)"=w439, "Channels data"=w449, "Channels config"=T4 [{"Name"="Z (m)", "Calibration"=1.0, "Offset"=0.0, "Channel index"=0}], "Filename control"=w440) -> ("error out"=w417:errorcluster)  [unwired: 2 in, 2 out]
        n193 = Strip Path(path=w412) -> (stripped path=w419:path)  [unwired: 1 out]
        n194 = Strip Path(path=w419) -> (stripped path=w393:path)  [unwired: 1 out]
        n195 = call <userlib>:"Get Session Path.vi"("error in (no error)"=w417, "Application ref in"=w416) -> ("error out"=w413:errorcluster, "Session path"=w415:path, "Application ref out"=w397:refnum<vi>)  [unwired: 7 in]
        n196 = Path To String(path=w412) -> (string=w411:string)
        n197 = call "SXM.vi"("Path"=w415, "Delete"=FALSE, "error in"=w413) -> ("error out"=w395:errorcluster)  [unwired: 7 in]
        n198 = call <userlib>:"Set Session Path.vi"("Save settings to previous? (False)"=TRUE, "error in (no error)"=w395, "Session Folder"=w393, "Application ref in"=w397) -> ("error out"=w394:errorcluster, "Application ref out"=w396:refnum<vi>)  [unwired: 6 in]
        n199 = Format Date/Time String(time format string (%c)=" Finished at %y%m%d - %H%M%S ", seconds (now)=w408) -> (date/time string=w407:string)  [unwired: 1 in]
        n200 = Concatenate Strings(w411, "\r\n", w407) -> (w410:string)
        n201 = Search and Replace String(input string="Email when finished", search string="@") -> (number of replacements=w403:i32)  [unwired: 6 in, 3 out]
        n202 = Greater Than 0?(x=w403) -> (x > 0?=w402:bool)
        n203 = case shown="True" w402 {
          tunnel: w394 -> [_ w457]
          tunnel: w410 -> [_ w455]
          tunnel: "Email when finished" -> [_ w454]
          frame False {
          }
          frame True {
            n204 = call "Send Email"("error in"=w457, "Message"=w455, "Subject"="Grid Finished", "Recipients"=w454) -> ()  [unwired: 7 in, 1 out]
          }
        }
        n205 = call <userlib>:"BiasSpectroscopy SetProperties.vi"("Application ref in"=w396, "Z-Controller hold (no change)"=enum16{"no change", "on", "off"}."on") -> ("Application ref out"=w400:refnum<vi>)  [unwired: 12 in, 1 out]
        n206 = call <userlib>:"TipLift Set.vi"("TipLift (m)"=sgl 0.0, "Application ref in"=w400) -> ("Application ref out"=w399:refnum<vi>)  [unwired: 8 in, 1 out]
      }
    }
    "Error out" <- w43
    "Points taken" <- w11
    "X Offset" <- w10
    "Y Offset" <- w9
  }
